vi "ams_demo (1).vi"() -> ()   [LabVIEW 2017]
uses:
  <vilib>/Instr/_visa.llb/VISA Configure Serial Port (Instr).vi
  <vilib>/Utility/file.llb/Write Delimited Spreadsheet (DBL).vi
panel:
  in  "采样率（个数/秒）":enum16{"6/s", "5/s", "1/s", "1/2s"}(ring)
  in  "保存按钮":bool
  in  "确定按钮":bool
  in  "选项卡控件":enum32{"模式1", "模式2"}(tab)
  in  "SV":i32 min=0 max=100
  in  "SV_Lower":i16 min=0 max=250
  in  "L_Duration (min)":i16
  in  "SV_Upper":i16 min=0 max=250
  in  "U_Duration (min）":i16
  in  "file path (dialog if empty)":path caption="文件保存路径"
  in  "停止按钮":bool
  in  "当前通道":enum32{"模拟通道1"}(radio) caption="单选按钮"
  out "波形图":dbl[](graph)
  out "当前采样值":dbl(knob) scale=0.0..250.0
  in  "串口号：":refnum<visa-resource-name>
  # "基于Arduino+LabVIEW的多路数据采集系统"
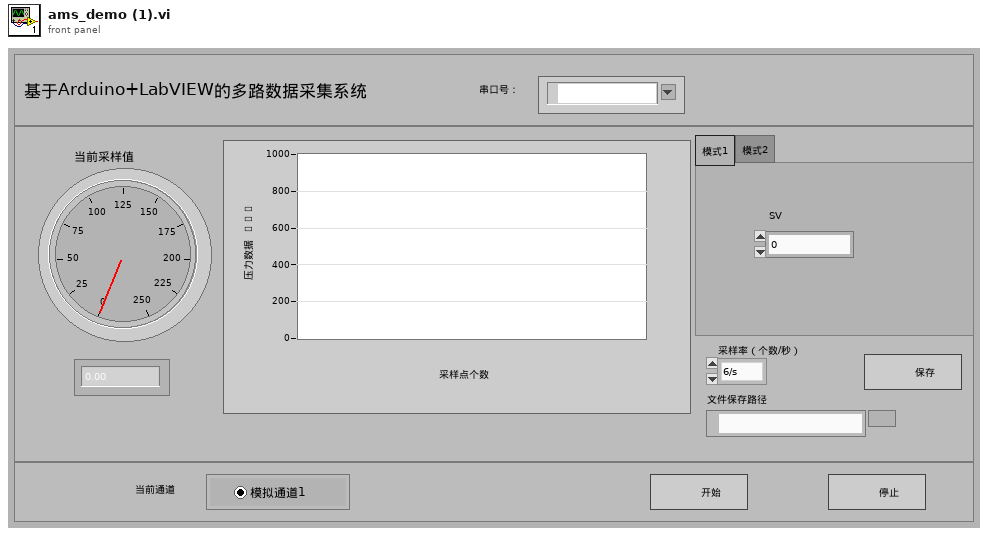
[diagram p1: front panel]
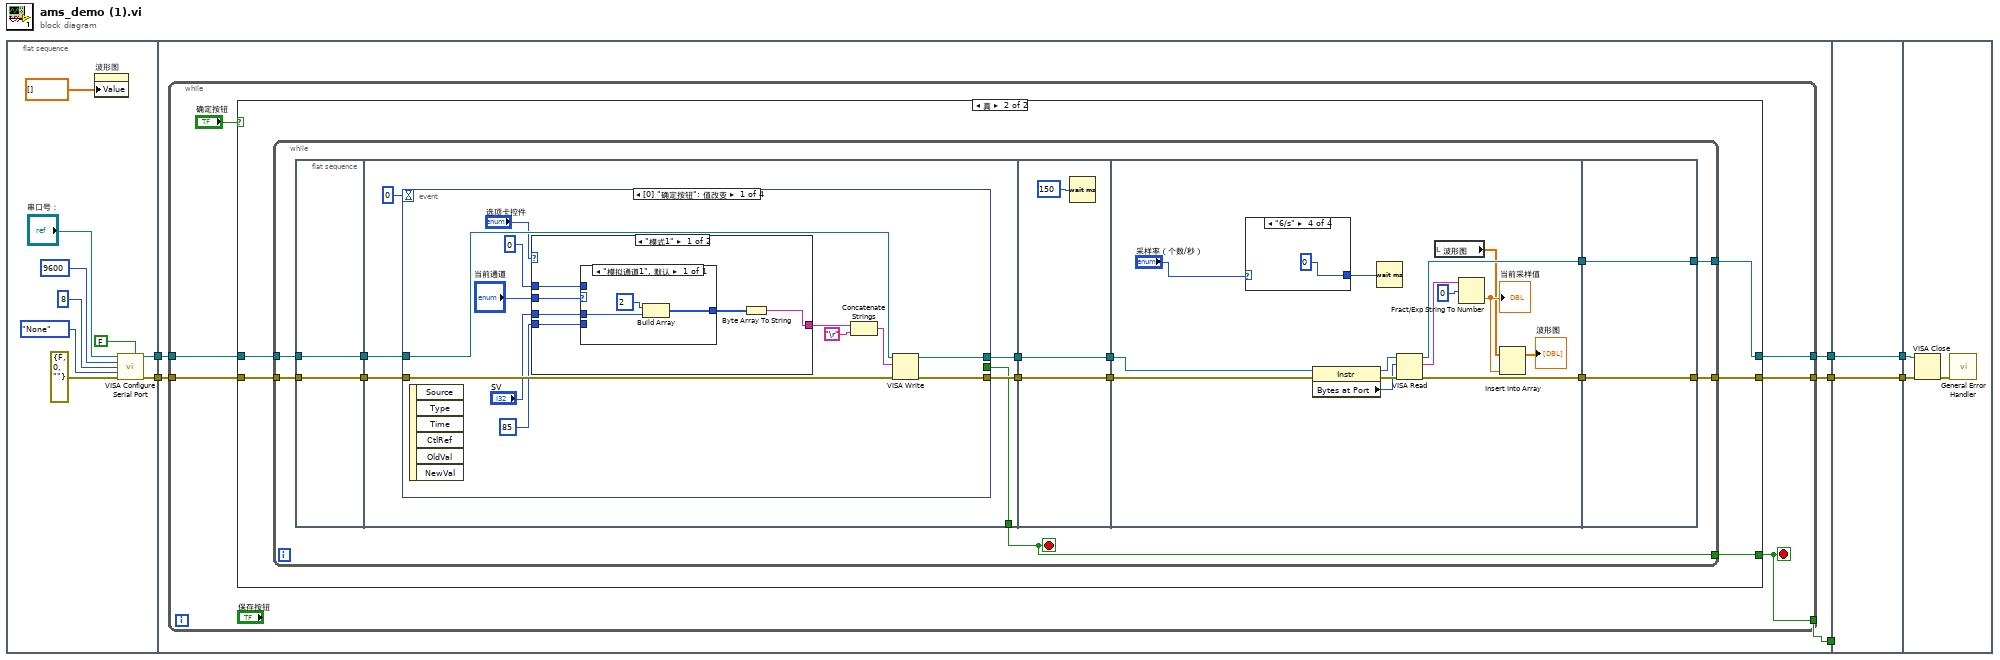
[diagram p0: block diagram]
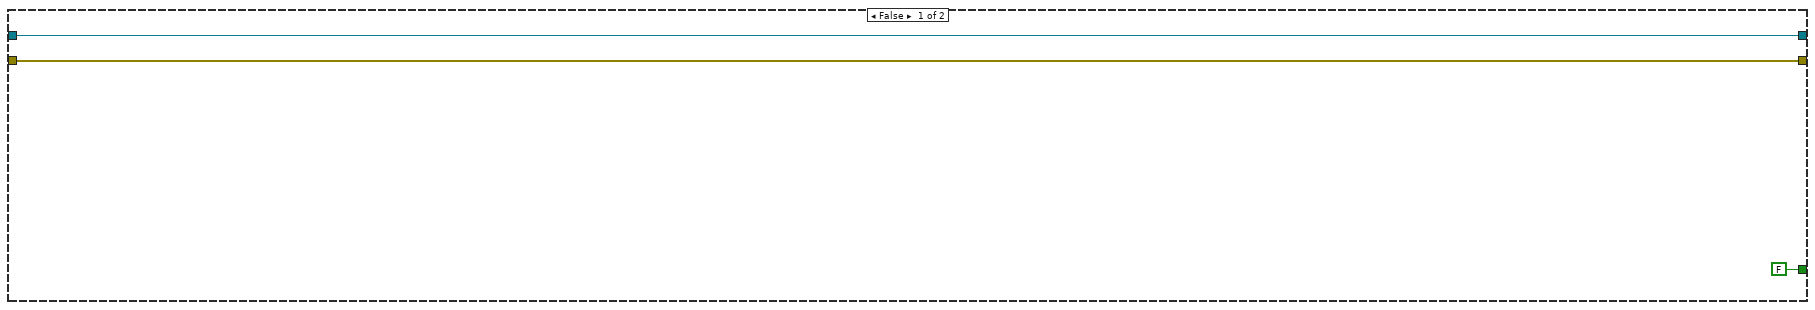
[diagram p2: hidden frame]
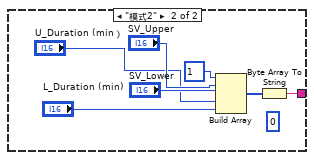
[diagram p3: hidden frame]
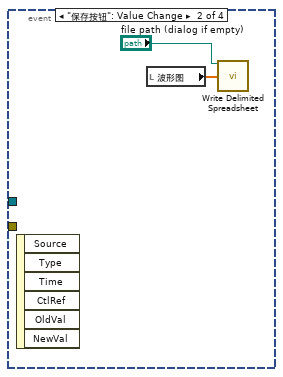
[diagram p4: hidden frame]
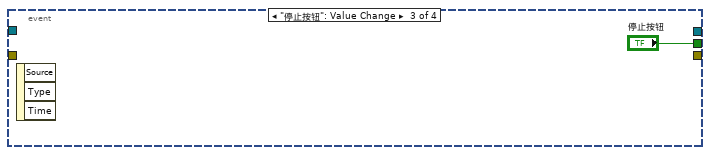
[diagram p5: hidden frame]
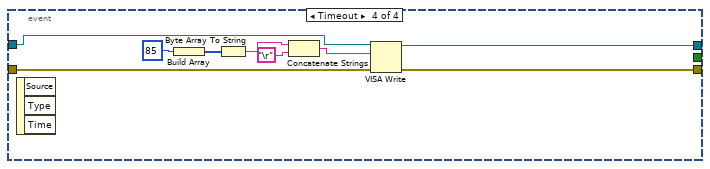
[diagram p6: hidden frame]
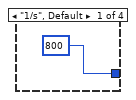
[diagram p7: hidden frame]
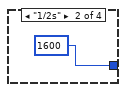
[diagram p8: hidden frame]
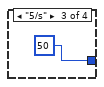
[diagram p9: hidden frame]
diagram:
  n1 = flat-sequence {
    tunnel: [w10] -> w7
    tunnel: [w9] -> w6
    tunnel: w7 -> [w21]
    tunnel: w6 -> [w20]
    tunnel: [w19] -> w5
    tunnel: [w18] -> w3
    tunnel: [w17] -> w1
    tunnel: w5 -> [w121]
    tunnel: [w121] -> w4
    tunnel: w3 -> [w120]
    tunnel: [w120] -> w2
    tunnel: w1 -> [_]
    tunnel: w4 -> [w123]
    tunnel: w2 -> [w122]
    frame #0 {
      n2 = property on="波形图" class="WFGraph (严格)"("Value"=dbl[] [] ("波形图")) -> ()  [unwired: 2 in, 2 out]
      n3 = call-poly "VISA Configure Serial Port"("VISA resource name"="串口号：", "Enable Termination\nChar (T)"=FALSE ("Enable Termination\nChar (T)"), "baud rate (9600)"=u32 9600, "data bits (8)"=u16 8, "parity (0:none)"=enum16{"None", "Odd", "Even", "Mark", "Space"}."None", "error in (no error)"=errorcluster {"status"=FALSE, "code"=0, "source"=""}) -> ("VISA resource name out"=w10:refnum<visa-resource-name>, "error out"=w9:errorcluster)  [unwired: 1 in, 7 out]
    }
    frame #1 {
      n4 = while {
        tunnel: w21 -> [w27]
        tunnel: w20 -> [w26]
        tunnel: [w25] -> w19
        tunnel: [w24] -> w18
        tunnel: [w23] -> w17
        stop <- w23 stop-if-true
        n5 = case shown="真" "确定按钮" {
          tunnel: w27 -> [w29 w35]
          tunnel: w26 -> [w28 w34]
          tunnel: [w29 w33] -> w25
          tunnel: [w28 w32] -> w24
          tunnel: [FALSE ("停止按钮") w31] -> w23
          frame False {
          }
          frame True {
            n6 = while {
              tunnel: [w36] -> w31
              tunnel: w35 -> [w40]
              tunnel: [w38] -> w33
              tunnel: w34 -> [w39]
              tunnel: [w37] -> w32
              stop <- w36 stop-if-true
              n7 = flat-sequence {
                tunnel: w39 -> [w49]
                tunnel: w40 -> [w50]
                tunnel: [w50] -> w48
                tunnel: [w49] -> w47
                tunnel: [w56] -> w46
                tunnel: [w55] -> w45
                tunnel: [w52] -> w36
                tunnel: w48 -> [w53]
                tunnel: w47 -> [w54]
                tunnel: w46 -> [w99]
                tunnel: w45 -> [w98]
                tunnel: [w99] -> w44
                tunnel: [w98] -> w43
                tunnel: w44 -> [w103]
                tunnel: w43 -> [w102]
                tunnel: [w111] -> w42
                tunnel: [w110] -> w41
                tunnel: w42 -> [w119]
                tunnel: w41 -> [w118]
                tunnel: [w119] -> w38
                tunnel: [w118] -> w37
                frame #0 {
                }
                frame #1 {
                  n8 = event shown="[0] \"确定按钮\": 值改变" {
                    selector: _ -> [_ _ _ _]
                    dyn-events: _ -> [_ _ _ _]
                    timeout: 0 -> [_ _ _ _]
                    tunnel: [w68 _ _ w89] -> w56
                    tunnel: [w67 _ _ w88] -> w55
                    tunnel: w54 -> [w66 _ _ w90]
                    tunnel: w53 -> [w65 _ _ w91]
                    tunnel: [_ _ "停止按钮" _] -> w52
                    event "确定按钮": Value Change {
                      n9 = event-data() -> ()  [unwired: 1 in, 6 out]
                      n10 = case shown="\"模式1\"" "选项卡控件" {
                        tunnel: "当前通道" -> [w74 _]
                        tunnel: "SV" -> [w72 _]
                        tunnel: i8 85 -> [w73 _]
                        tunnel: i16 0 -> [w71 _]
                        tunnel: [w69 w82] -> w57
                        frame "模式1" {
                          n11 = case shown="\"模拟通道1\", 默认" w74 {
                            tunnel: [w77] -> w70
                            tunnel: w73 -> [_]
                            tunnel: w72 -> [w75]
                            tunnel: w71 -> [_]
                            frame "模拟通道1", Default {
                              n12 = Build Array(i16 2, w75) -> (w77:i32[])
                            }
                          }
                          n13 = Byte Array To String(unsigned byte array=w70) -> (string=w69:string)
                        }
                        frame "模式2" {
                          (unwired) i16 0 ("元素")
                          n14 = Build Array(i8 1, "SV_Upper", "SV_Lower", "U_Duration (min）", "L_Duration (min)") -> (w83:i16[])
                          n15 = Byte Array To String ("字节数组至字符串转换")(unsigned byte array=w83) -> (string=w82:string)
                        }
                      }
                      n16 = Concatenate Strings(w57, "\r") -> (w63:string)
                      n17 = VISA Write(VISA resource name=w65, write buffer=w63, error in (no error)=w66) -> (VISA resource name out=w68:refnum<visa-resource-name>, error out=w67:errorcluster)  [unwired: 1 out]
                    }
                    event "保存按钮": Value Change {
                      n18 = event-data() -> ()  [unwired: 1 in, 6 out]
                      n19 = local read "波形图"() -> (w86:dbl[])
                      n20 = call-poly <vilib>:"Write Delimited Spreadsheet.vi"("file path (dialog if empty)"="file path (dialog if empty)", "1D data"=w86) -> ()  [unwired: 12 in, 2 out]
                    }
                    event "停止按钮": Value Change {
                      n21 = event-data() -> ()  [unwired: 1 in, 3 out]
                    }
                    event Timeout {
                      n22 = event-data() -> ()  [unwired: 1 in, 3 out]
                      n23 = Build Array(i16 85) -> (w92:i16[])
                      n24 = Byte Array To String(unsigned byte array=w92) -> (string=w96:string)
                      n25 = Concatenate Strings(w96, "\r") -> (w94:string)
                      n26 = VISA Write(VISA resource name=w91, write buffer=w94, error in (no error)=w90) -> (VISA resource name out=w89:refnum<visa-resource-name>, error out=w88:errorcluster)  [unwired: 1 out]
                    }
                  }
                }
                frame #2 {
                  n27 = Wait (ms)(milliseconds to wait=u32 150 ("等待时间（毫秒）")) -> ()  [unwired: 1 out]
                }
                frame #3 {
                  n28 = case shown="\"6/s\"" "采样率（个数/秒）" {
                    tunnel: [800 1600 50 0] -> w100
                    frame "1/s", Default {
                    }
                    frame "1/2s" {
                    }
                    frame "5/s" {
                    }
                    frame "6/s" {
                    }
                  }
                  n29 = property class="Instr"(reference=w103, error in=w102) -> (reference out=w108:refnum<visa-resource-name>, error out=w107:errorcluster, "Bytes at Port"=w106:u32)
                  n30 = Wait (ms)(milliseconds to wait=w100) -> ()  [unwired: 1 out]
                  n31 = VISA Read(VISA resource name=w108, byte count=w106, error in (no error)=w107) -> (VISA resource name out=w111:refnum<visa-resource-name>, read buffer=w109:string, error out=w110:errorcluster)  [unwired: 1 out]
                  n32 = local read "波形图"() -> (w104:dbl[])
                  n33 = Fract/Exp String To Number(string=w109, offset=0 ("偏移量")) -> (number=w112:dbl)  [unwired: 2 in, 1 out]
                  "当前采样值" <- w112
                  n34 = Insert Into Array(array=w104, new element=w112) -> (→"波形图":dbl[])  [unwired: 1 in]
                }
                frame #4 {
                }
              }
            }
          }
        }
      }
    }
    frame #2 {
    }
    frame #3 {
      n35 = VISA Close(VISA resource name=w123, error in (no error)=w122) -> (error out=w124:errorcluster)
      n36 = call <vilib>:"General Error Handler.vi"("error in (no error)"=w124) -> ()  [unwired: 10 in, 5 out]
    }
  }
